vi "Auto Power Spectrum PtByPt.vi"(0 "signal":dbl format="%0.2f", 1 "sample length":i32=100, 2 "dt":dbl=1.0 format="%0.2f", 4 "initialize":bool) -> (5 "Power Spectrum (V^2 rms)":dbl[](array[numeric]), 6 "df":dbl format="%0.2f", 7 "error":i32)   [LabVIEW 2020, in "NI_PtbyPt.lvlib"]
doc: "Computes the single-sided, scaled, auto power spectrum of a time-domain <B>signal</B>."
uses:
  NI_PtbyPt.lvlib
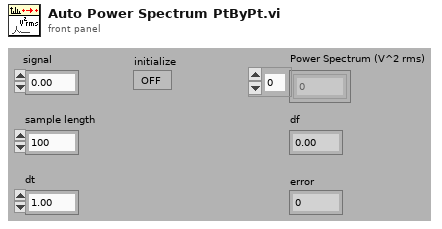
[diagram p1: front panel]
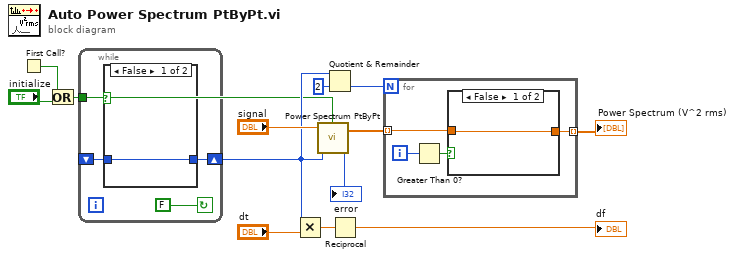
[diagram p0: block diagram]
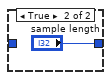
[diagram p2: hidden frame]
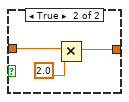
[diagram p3: hidden frame]
diagram:
  n1 = First Call?() -> (First Call?: T/F=w1:bool)
  n2 = Or(x=w1, y="initialize") -> (x .or. y?=w3:bool)
  n3 = while {
    shift-left: _ -> [w15]
    shift-right: [w16] -> w4
    tunnel: w3 -> [w17]
    stop <- FALSE continue-if-true
    n4 = case shown="False" w17 {
      tunnel: [w18 "sample length"] -> w16
      tunnel: w15 -> [w18 _]
      frame False {
      }
      frame True {
      }
    }
  }
  n5 = Multiply(x=w4, y="dt") -> (x*y=w13:dbl)
  n6 = call "Power Spectrum PtByPt.vi"("initialize"=w3, "sample length"=w4, "x"="signal") -> ("error"=→"error":i32, "Power Spectrum"=w9:dbl[])  [unwired: 1 in]
  n7 = Quotient & Remainder(x=w4, y=2) -> (floor(x/y)=w6:i32)  [unwired: 1 out]
  n8 = Reciprocal(x=w13) -> (1/x=→"df":dbl)
  n9 = for {
    N: w6 -> [_]
    tunnel: [w21] -> w10 mode=indexing
    tunnel: w9 -> [w20] mode=indexing
    i -> [w23]
    n10 = Greater Than 0?(x=w23) -> (x > 0?=w22:bool)
    n11 = case shown="False" w22 {
      tunnel: [w24 w27] -> w21
      tunnel: w20 -> [w24 w26]
      frame False {
      }
      frame True {
        n12 = Multiply(x=w26, y=2.0) -> (x*y=w27:dbl)
      }
    }
  }
  "Power Spectrum (V^2 rms)" <- w10
